vi "query(byVal).vi"(6 "use Regex? (F)":bool, 9 "Search string":string, 10 "Search Key (FQN)":T1, 11 "Instance":refnum<class "NameRegistry.lvclass">) -> (1 "Nodes":refnum<class "UniqueName.lvclass">[](array[class]), 2 "First Node":refnum<class "UniqueName.lvclass">, 3 "Instance":refnum<class "NameRegistry.lvclass">, 4 "found?":bool)   [LabVIEW 2014, in "UniqueName.lvlib" / "NameRegistry.lvclass"]
uses:
  NameRegistry.lvclass
  UniqueNameClass/Key.ctl
  UniqueNameClass/UniqueName.lvclass
  NameRegistry.lvclass/NameRegistry.ctl
  UniqueNameClass/UniqueName.lvclass/UniqueName.ctl
  <vilib>/regexp/Match Regular Expression.xnode
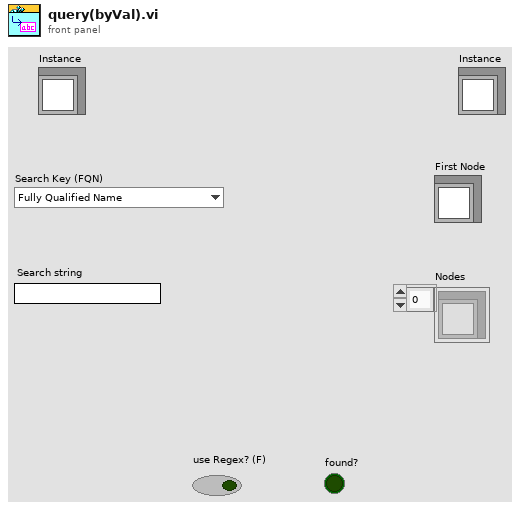
[diagram p1: front panel]
types:
  T1 = typedef "UniqueName.lvlib/UniqueName.lvclass/Key.ctl" = enum16{"Fully Qualified Name", "Unique Name", "Given Name", "Parent Fully Qualified Name"}
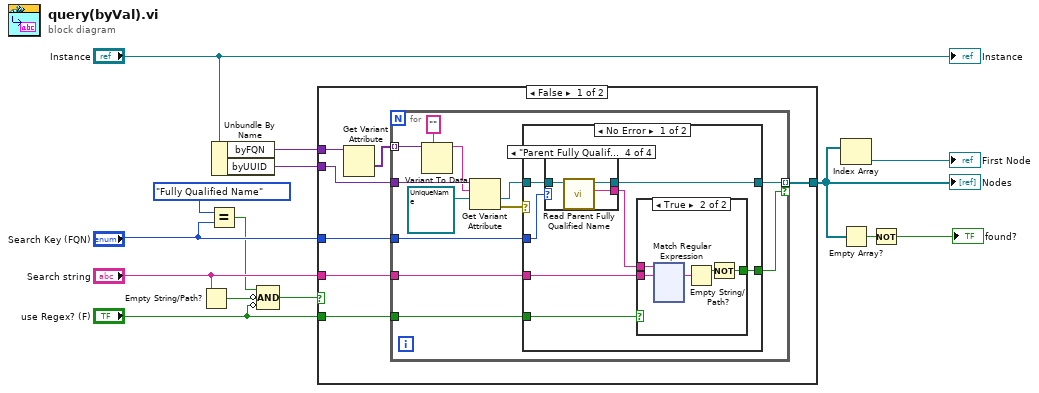
[diagram p0: block diagram]
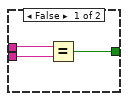
[diagram p2: hidden frame]
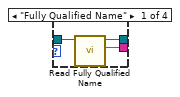
[diagram p3: hidden frame]
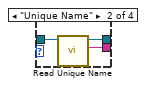
[diagram p4: hidden frame]
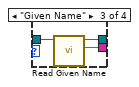
[diagram p5: hidden frame]
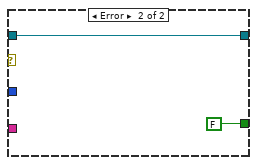
[diagram p6: hidden frame]
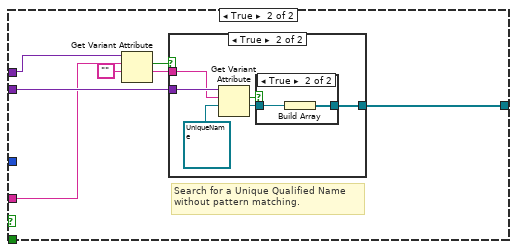
[diagram p7: hidden frame]
diagram:
  n1 = Empty String/Path?(string/path="Search string") -> (empty?=w5:bool)
  n2 = Equal?(x=Key."Fully Qualified Name", y="Search Key (FQN)") -> (x = y?=w6:bool)
  n3 = Unbundle By Name("Instance") -> ("byFQN"=w4:variant, "byUUID"=w3:variant)
  n4 = Compound Arithmetic op=AND(w6, invert w5, invert "use Regex? (F)") -> (w2:bool)
  n5 = case shown="False" w2 {
    tunnel: w3 -> [w16 w183]
    tunnel: [w21 w182] -> w10
    tunnel: "Search string" -> [w19 w180]
    tunnel: "Search Key (FQN)" -> [w18 _]
    tunnel: "use Regex? (F)" -> [w20 _]
    tunnel: w4 -> [w17 w177]
    frame False {
      n6 = Get Variant Attribute(Variant=w17) -> (values=w15:variant[])  [unwired: 3 in, 3 out]
      n7 = for {
        tunnel: w16 -> [w28]
        tunnel: [w32] -> w21 mode=indexing if=w31
        tunnel: w20 -> [w30]
        tunnel: w19 -> [w29]
        tunnel: w18 -> [w33]
        tunnel: w15 -> [w27] mode=indexing
        n8 = Variant To Data(type="", Variant=w27) -> (data=w25:string)  [unwired: 1 in, 1 out]
        n9 = Get Variant Attribute(Variant=w28, name=w25, default value (empty Variant)=refnum<class "UniqueName.lvclass"> refnum ("UniqueName.lvclass")) -> (value=w23:refnum<class "UniqueName.lvclass">, error out=w22:errorcluster)  [unwired: 1 in, 2 out]
        n10 = case shown="No Error" w22 {
          tunnel: [w34 FALSE] -> w31
          tunnel: w33 -> [w40 _]
          tunnel: w23 -> [w39 w176]
          tunnel: [w38 w176] -> w32
          tunnel: w30 -> [w37 _]
          tunnel: w29 -> [w35 _]
          frame No Error {
            n11 = case shown="\"Parent Fully Qualified Name\"" w40 {
              tunnel: w39 -> [w165 w168 w171 w174]
              tunnel: [w164 w167 w170 w173] -> w38
              tunnel: [w163 w166 w169 w172] -> w36
              frame "Fully Qualified Name" {
                n12 = call "Read Fully Qualified Name.vi"("UniqueName in"=w165) -> ("Fully Qualified Name"=w163:string, "UniqueName out"=w164:refnum<class "UniqueName.lvclass">)  [unwired: 9 in]
              }
              frame "Unique Name" {
                n13 = call "Read Unique Name.vi"("UniqueName in"=w168) -> ("Unique Name"=w166:string, "UniqueName out"=w167:refnum<class "UniqueName.lvclass">)  [unwired: 9 in]
              }
              frame "Given Name" {
                n14 = call "Read Given Name.vi"("UniqueName in"=w171) -> ("Given Name"=w169:string, "UniqueName out"=w170:refnum<class "UniqueName.lvclass">)  [unwired: 9 in]
              }
              frame "Parent Fully Qualified Name" {
                n15 = call "Read Parent Fully Qualified Name.vi"("UniqueName in"=w174) -> ("Parent Fully Qualified Name"=w172:string, "UniqueName out"=w173:refnum<class "UniqueName.lvclass">)  [unwired: 9 in]
              }
            }
            n16 = case shown="True" w37 {
              tunnel: w36 -> [w43 w48]
              tunnel: w35 -> [w42 w47]
              tunnel: [w41 w44] -> w34
              frame False {
                n17 = Equal?(x=w43, y=w42) -> (x = y?=w41:bool)
              }
              frame True {
                n18 = xnode "Match Regular Expression"("input string"=w48, "regular expression"=w47) -> ("whole match"=w46:string)  [unwired: 4 in, 4 out]
                n19 = Empty String/Path?(string/path=w46) -> (empty?=w45:bool)
                n20 = Not(x=w45) -> (.not. x?=w44:bool)
              }
            }
          }
          frame Error {
          }
        }
      }
    }
    frame True {
      # "Search for a Unique Qualified Name\nwithout pattern matching."
      n21 = Get Variant Attribute(Variant=w177, name=w180, default value (empty Variant)="") -> (found=w178:bool, value=w179:string)  [unwired: 1 in, 2 out]
      n22 = case shown="True" w178 {
        tunnel: w183 -> [_ w189]
        tunnel: [_ w187] -> w182
        tunnel: w179 -> [_ w185]
        frame False {
        }
        frame True {
          n23 = Get Variant Attribute(Variant=w189, name=w185, default value (empty Variant)=refnum<class "UniqueName.lvclass"> refnum ("UniqueName Object (Set)")) -> (found=w186:bool, value=w188:refnum<class "UniqueName.lvclass">)  [unwired: 1 in, 2 out]
          n24 = case shown="True" w186 {
            tunnel: w188 -> [_ w191]
            tunnel: [_ w190] -> w187
            frame False {
            }
            frame True {
              n25 = Build Array(w191) -> (w190:refnum<class "UniqueName.lvclass">[])
            }
          }
        }
      }
    }
  }
  "Nodes" <- w10
  n26 = Index Array(array=w10) -> (element=→"First Node":refnum<class "UniqueName.lvclass">)  [unwired: 1 in]
  n27 = Empty Array?(array=w10) -> (empty?=w1:bool)
  n28 = Not(x=w1) -> (.not. x?=→"found?":bool)
  "Instance" <- "Instance"
